vi "PXI-6229Loop.vi"(8 "Error In":errorcluster, 9 "ABLE Configuration":T1, 10 "PXI-6229 Data Notifier":refnum<notifier>, 11 "PXI-6229 Action Queue":refnum<queue>) -> (0 "Error Out":errorcluster)   [LabVIEW 2012]
uses:
  PXI6229ActionQueueElement.ctl
  PXI6229Action.ctl
  ABLEConfiguration.ctl
  DisplayConfiguration.ctl
  FolderConfiguration.ctl
  AlarmsConfiguration.ctl
  Keithley6485Configuration.ctl
  Keithley6482Configuration.ctl
  PXI6229Data.ctl
  <vilib>/Utility/error.llb/DialogType.ctl
  libs/LV-Utilities/LV-Utilities.lvlib
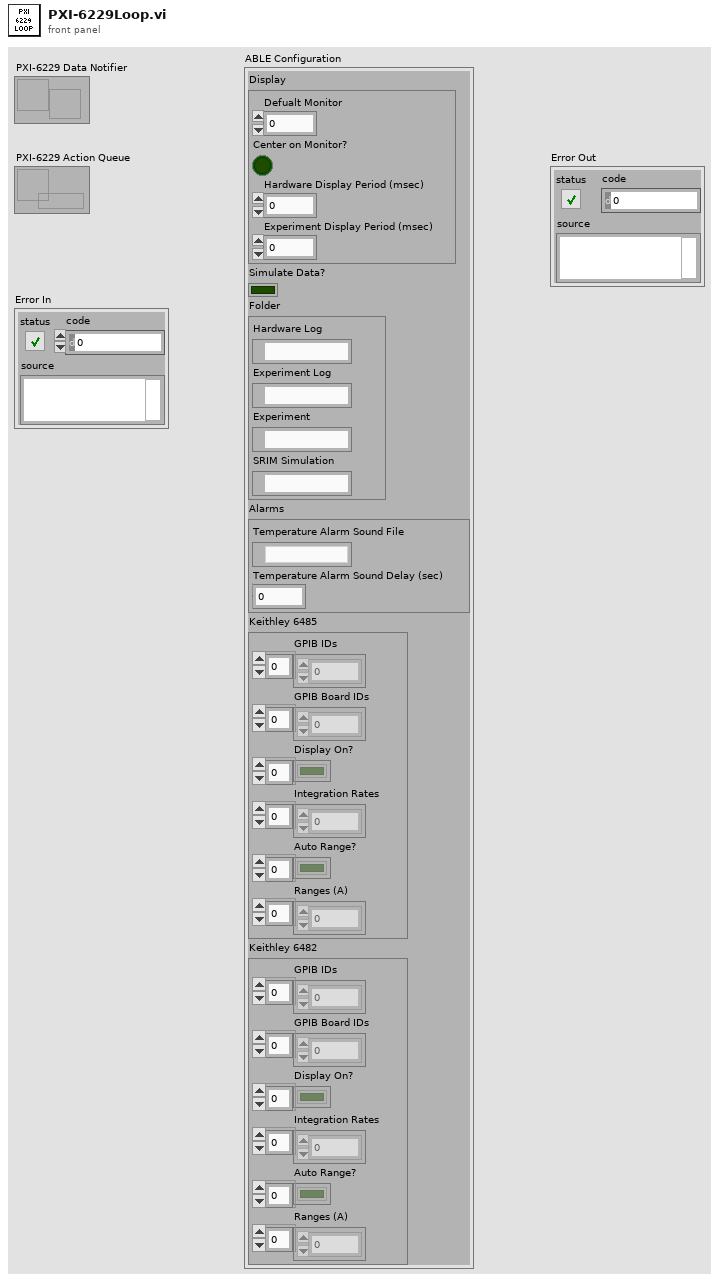
[diagram p1: front panel]
types:
  T1 = typedef "ABLEConfiguration.ctl" = cluster{"Display":T2, "Simulate Data?":bool, "Folder":T3, "Alarms":T4, "Keithley 6485":T5, "Keithley 6482":T6}
  T2 = typedef "DisplayConfiguration.ctl" = cluster{"Defualt Monitor":u16, "Center on Monitor?":bool, "Hardware Display Period (msec)":u32, "Experiment Display Period (msec)":u32}
  T3 = typedef "FolderConfiguration.ctl" = cluster{"Hardware Log":path, "Experiment Log":path, "Experiment":path, "SRIM Simulation":path}
  T4 = typedef "AlarmsConfiguration.ctl" = cluster{"Temperature Alarm Sound File":path, "Temperature Alarm Sound Delay (sec)":dbl}
  T5 = typedef "Keithley6485Configuration.ctl" = cluster{"GPIB IDs":u8[], "GPIB Board IDs":u8[], "Display On?":bool[], "Integration Rates":dbl[], "Auto Range?":bool[], "Ranges (A)":dbl[]}
  T6 = typedef "Keithley6482Configuration.ctl" = cluster{"GPIB IDs":u8[], "GPIB Board IDs":u8[], "Display On?":bool[], "Integration Rates":dbl[], "Auto Range?":bool[], "Ranges (A)":dbl[]}
  T7 = typedef "PXI6229Data.ctl" = cluster{"Temperatures":dbl[][], "Terminal Voltage":dbl[][], "BPM":dbl[][]}
  T8 = typedef "PXI6229ActionQueueElement.ctl" = cluster{"Action":T9, "Data":variant}
  T9 = typedef "PXI6229Action.ctl" = enum16{"Initialize", "Read", "Simulate", "Error", "Shutdown"}
  T10 = typedef "DialogType.ctl" = u16
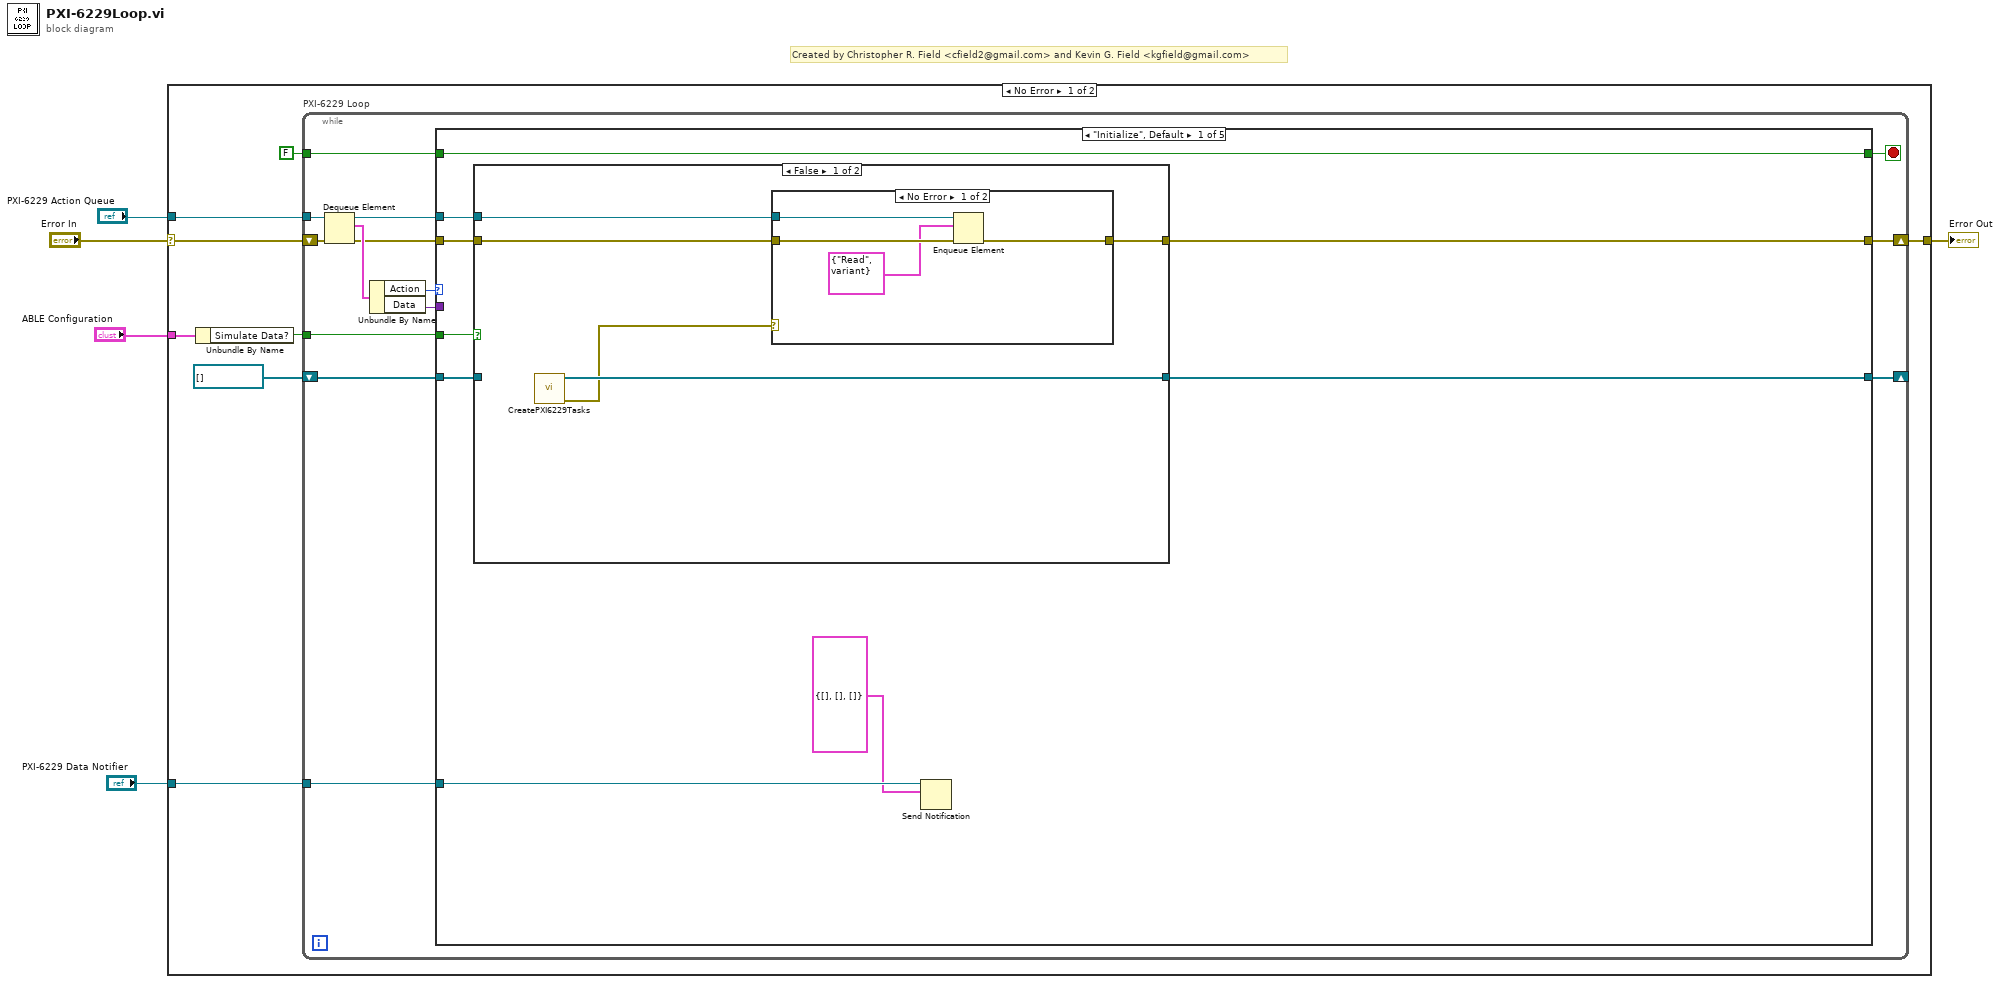
[diagram p0: block diagram]
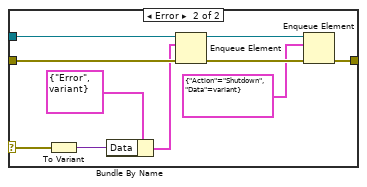
[diagram p2: hidden frame]
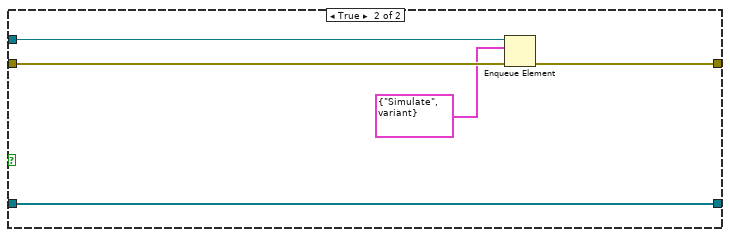
[diagram p3: hidden frame]
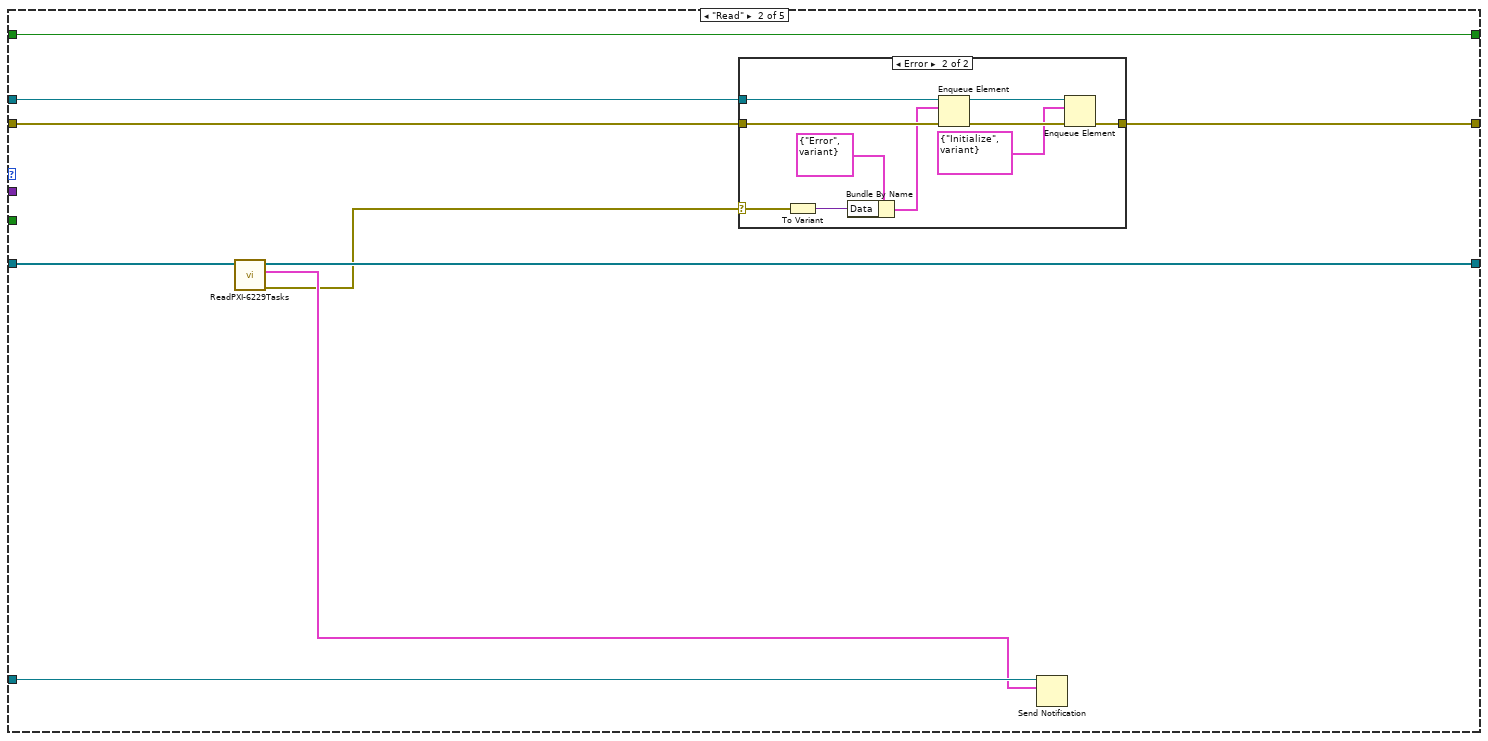
[diagram p4: hidden frame]
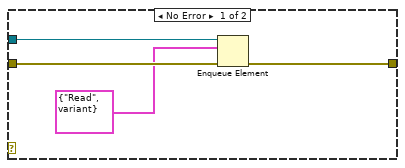
[diagram p5: hidden frame]
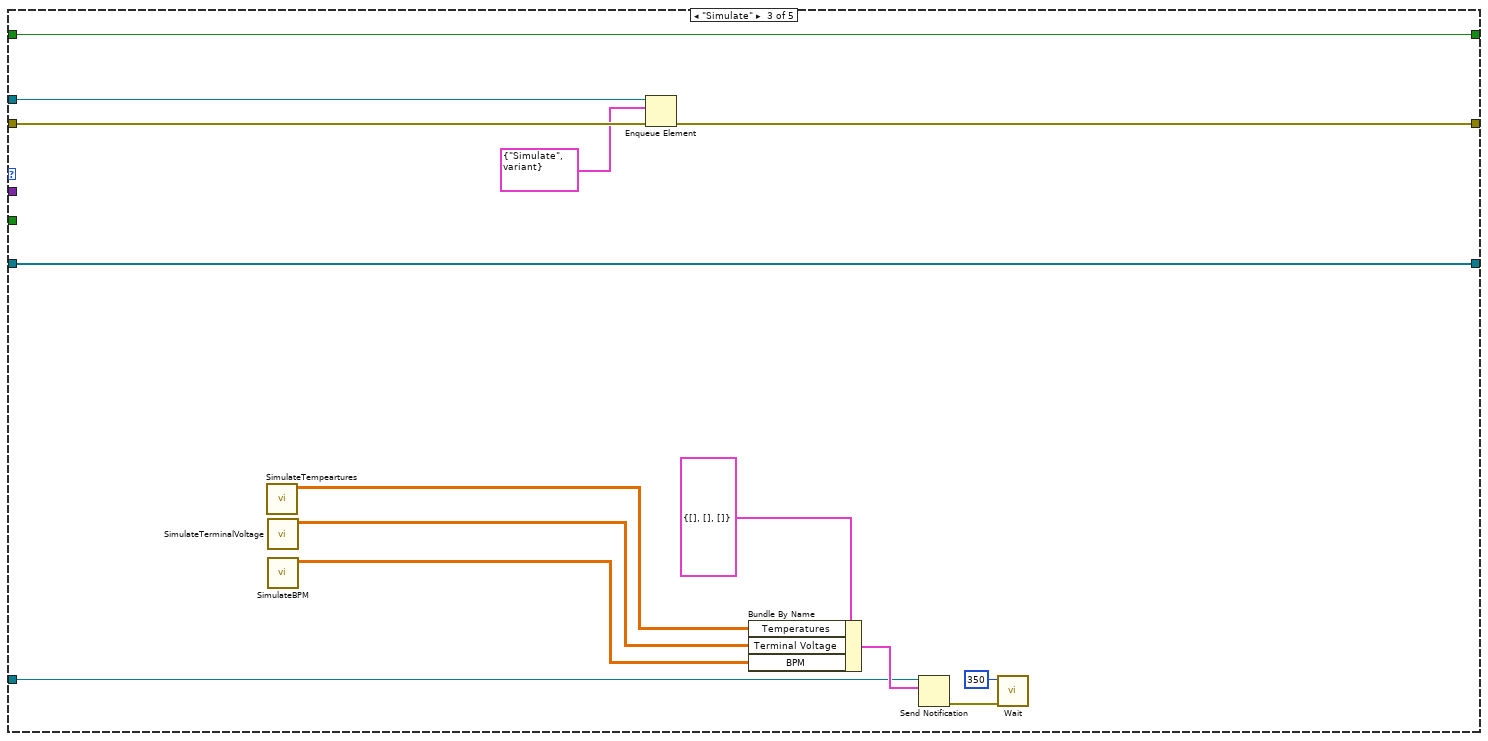
[diagram p6: hidden frame]
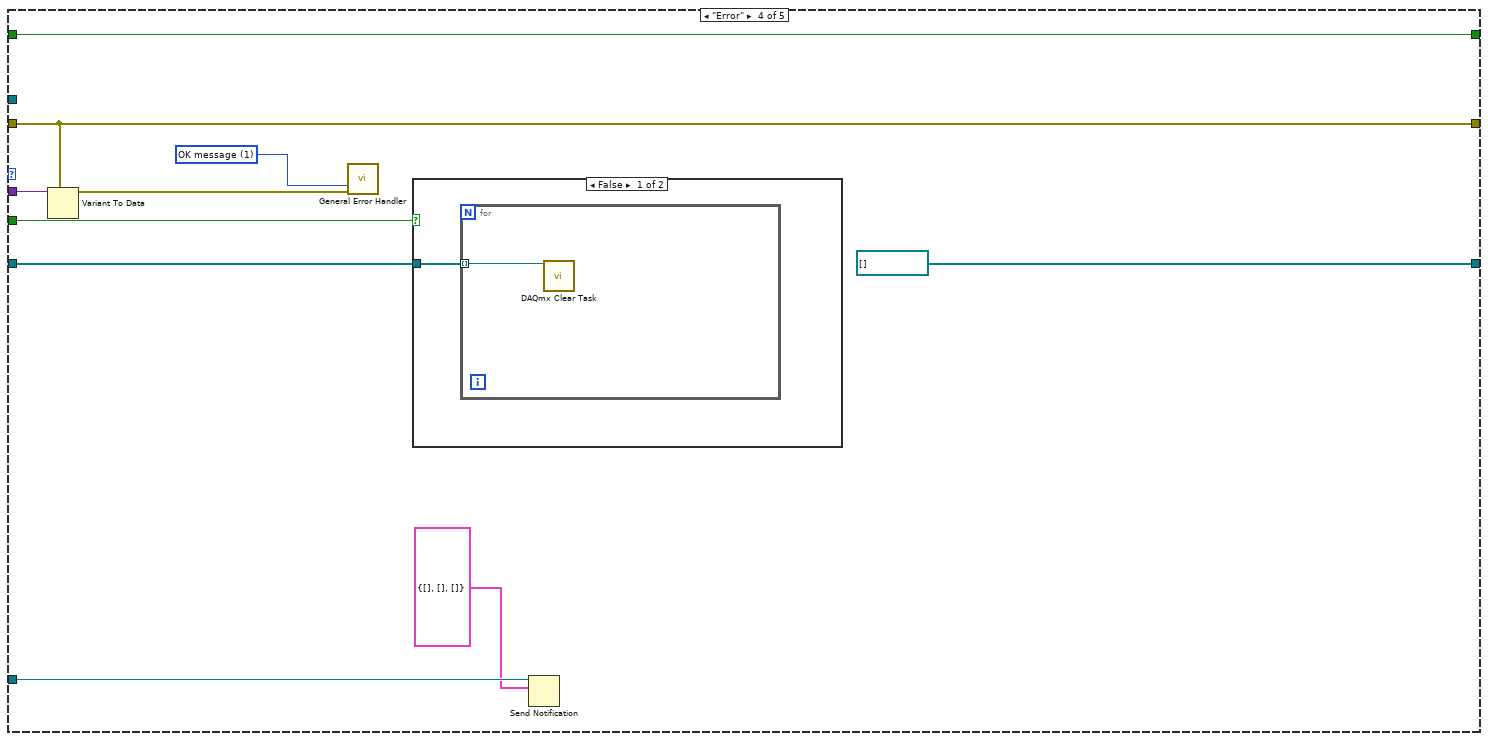
[diagram p7: hidden frame]
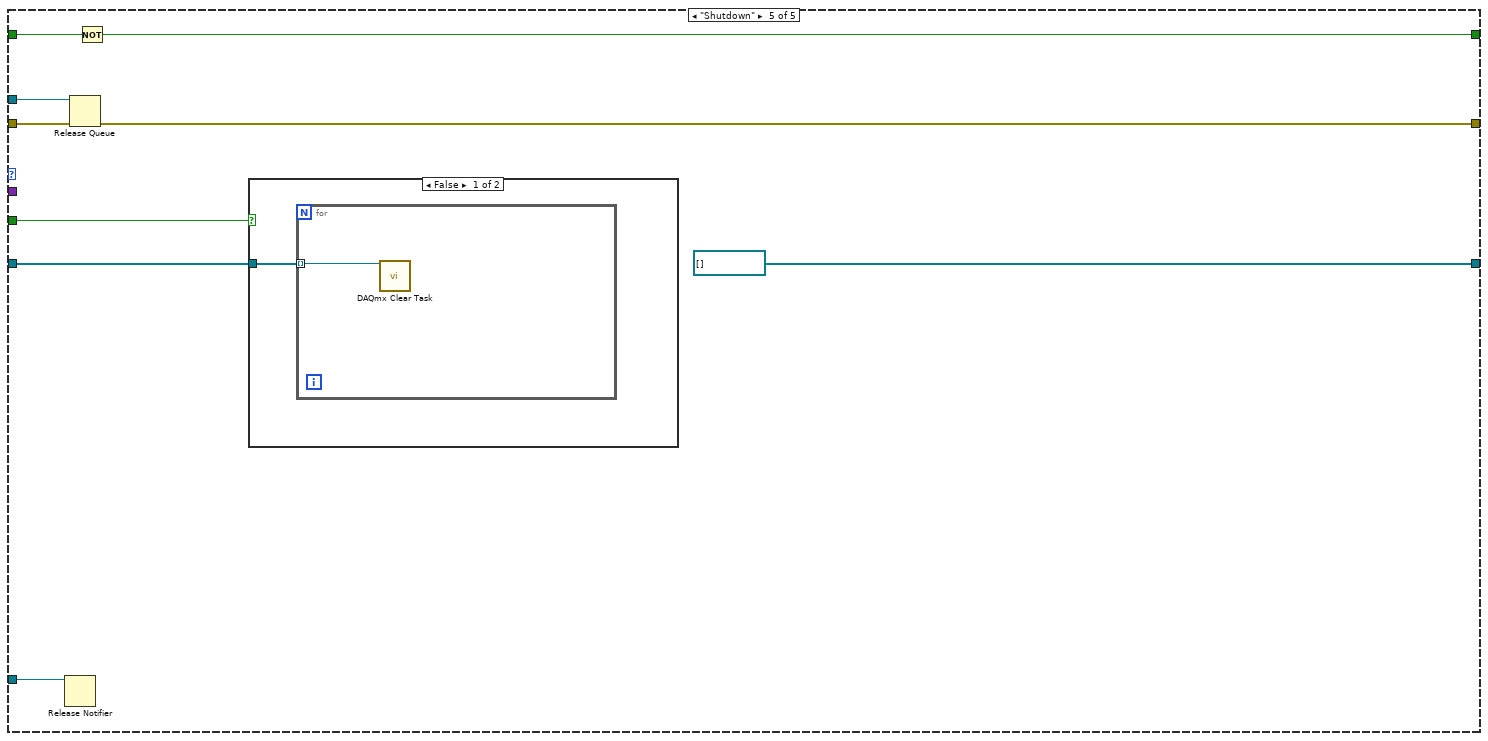
[diagram p9: hidden frame]
diagram:
  # "Created by Christopher R. Field <cfield2@gmail.com> and Kevin G. Field <kgfield@gmail.com>"
  n1 = case shown="No Error" "Error In" {
    selector: "Error In" -> [w10 w121]
    tunnel: "PXI-6229 Action Queue" -> [w13 _]
    tunnel: [w9 w121] -> w4
    tunnel: "PXI-6229 Data Notifier" -> [w11 _]
    tunnel: "ABLE Configuration" -> [w8 _]
    frame No Error {
      n2 = Unbundle By Name(w8) -> ("Simulate Data?"=w7:bool)
      n3 = while "PXI-6229 Loop" {
        tunnel: FALSE -> [w27]
        tunnel: w13 -> [w26]
        shift-right: [w18] -> w9
        shift-left: w10 -> [w25]
        tunnel: w11 -> [w17]
        shift-right: [w16] -> _
        shift-left: refnum<k21>[] [] -> [w15]
        tunnel: w7 -> [w14]
        stop <- w20 stop-if-true
        n4 = Dequeue Element(queue=w26, error in (no error)=w25) -> (queue out=w21:refnum<queue>, element=w24:T8, error out=w22:errorcluster)  [unwired: 1 in, 1 out]
        n5 = Unbundle By Name(w24) -> ("Action"=w23:T9, "Data"=w19:variant)
        n6 = case shown="\"Initialize\", Default" w23 {
          tunnel: w27 -> [w36 w69 w94 w107 w118]
          tunnel: w22 -> [w34 w66 w96 w103 w114]
          tunnel: w21 -> [w33 w68 w97 _ w116]
          tunnel: [w36 w69 w94 w107 w117] -> w20
          tunnel: w19 -> [_ _ _ w106 _]
          tunnel: [w32 w67 w95 w103 w115] -> w18
          tunnel: w17 -> [w29 w65 w89 w102 w111]
          tunnel: [w35 w63 w93 refnum<k21>[] [] ("PXI-6229 Tasks Out") refnum<k21>[] [] ("PXI-6229 Tasks Out")] -> w16
          tunnel: w15 -> [w30 w64 w93 w100 w113]
          tunnel: w14 -> [w31 _ _ w99 w112]
          frame "Initialize", Default {
            n7 = case shown="False" w31 {
              tunnel: [w38 w60] -> w35
              tunnel: w34 -> [w41 w58]
              tunnel: w33 -> [w40 w59]
              tunnel: [w39 w57] -> w32
              tunnel: w30 -> [_ w60]
              frame False {
                n8 = call "CreatePXI6229Tasks.vi"() -> ("Error Out"=w37:errorcluster, "PXI-6229 Tasks Out"=w38:refnum<k21>[])  [unwired: 10 in]
                n9 = case shown="No Error" w37 {
                  selector: w37 -> [_ w52]
                  tunnel: w41 -> [w44 w54]
                  tunnel: w40 -> [w45 w55]
                  tunnel: [w43 w47] -> w39
                  frame No Error {
                    n10 = Enqueue Element(queue=w45, element=T8 {"Action"=enum."Read", "Data"=variant}, error in (no error)=w44) -> (error out=w43:errorcluster)  [unwired: 1 in, 2 out]
                  }
                  frame Error {
                    n11 = To Variant(anything=w52) -> (Variant=w51:variant)
                    n12 = Bundle By Name(cluster=T8 {"Action"=enum."Error", "Data"=variant} ("element"), "Data"=w51) -> (w50:T8)
                    n13 = Enqueue Element(queue=w55, element=w50, error in (no error)=w54) -> (queue out=w49:refnum<queue>, error out=w48:errorcluster)  [unwired: 1 in, 1 out]
                    n14 = Enqueue Element(queue=w49, element=T8 {"Action"=enum."Shutdown", "Data"=variant}, error in (no error)=w48) -> (error out=w47:errorcluster)  [unwired: 1 in, 2 out]
                  }
                }
              }
              frame True {
                n15 = Enqueue Element(queue=w59, element=T8 {"Action"=enum."Simulate", "Data"=variant}, error in (no error)=w58) -> (error out=w57:errorcluster)  [unwired: 1 in, 2 out]
              }
            }
            n16 = Send Notification(notification=T7 {"Temperatures"=[], "Terminal Voltage"=[], "BPM"=[]}, notifier=w29) -> ()  [unwired: 1 in, 2 out]
          }
          frame "Read" {
            n17 = call "ReadPXI-6229Tasks.vi"("PXI-6229 Tasks In"=w64) -> ("Error Out"=w61:errorcluster, "PXI-6229 Data"=w62:T7, "PXI-6229 Tasks Out"=w63:refnum<k21>[])  [unwired: 8 in]
            n18 = case shown="Error" w61 {
              selector: w61 -> [_ w80]
              tunnel: w68 -> [w73 w83]
              tunnel: [w72 w75] -> w67
              tunnel: w66 -> [w71 w82]
              frame No Error {
                n19 = Enqueue Element(queue=w73, element=T8 {"Action"=enum."Read", "Data"=variant}, error in (no error)=w71) -> (error out=w72:errorcluster)  [unwired: 1 in, 2 out]
              }
              frame Error {
                n20 = To Variant(anything=w80) -> (Variant=w79:variant)
                n21 = Bundle By Name(cluster=T8 {"Action"=enum."Error", "Data"=variant} ("element"), "Data"=w79) -> (w78:T8)
                n22 = Enqueue Element(queue=w83, element=w78, error in (no error)=w82) -> (queue out=w77:refnum<queue>, error out=w76:errorcluster)  [unwired: 1 in, 1 out]
                n23 = Enqueue Element(queue=w77, element=T8 {"Action"=enum."Initialize", "Data"=variant}, error in (no error)=w76) -> (error out=w75:errorcluster)  [unwired: 1 in, 2 out]
              }
            }
            n24 = Send Notification(notification=w62, notifier=w65) -> ()  [unwired: 1 in, 2 out]
          }
          frame "Simulate" {
            n25 = call "SimulateTempeartures.vi"() -> ("Simulated Temperatures"=w84:dbl[][])  [unwired: 11 in]
            n26 = call "SimulateTerminalVoltage.vi"() -> ("Simulated Terminal Voltage"=w88:dbl[][])  [unwired: 11 in]
            n27 = call "SimulateBPM.vi"() -> ("Simulated BPM"=w87:dbl[][])  [unwired: 11 in]
            n28 = Enqueue Element(queue=w97, element=T8 {"Action"=enum."Simulate", "Data"=variant}, error in (no error)=w96) -> (error out=w95:errorcluster)  [unwired: 1 in, 2 out]
            n29 = Bundle By Name(cluster=T7 {"Temperatures"=[], "Terminal Voltage"=[], "BPM"=[]} ("DAQ Data Queue Element"), "Temperatures"=w84, "Terminal Voltage"=w88, "BPM"=w87) -> (w90:T7)
            n30 = Send Notification(notification=w90, notifier=w89) -> (error out=w85:errorcluster)  [unwired: 1 in, 1 out]
            n31 = call "Wait.vi"("Error In"=w85, "Wait Time (msec)"=u32 350) -> ()  [unwired: 9 in, 1 out]
          }
          frame "Error" {
            w104 = T10 1 items=["no dialog", "OK message", "continue or stop message", "OK message + warnings", "continue/stop + warnings"] ("type of dialog (OK msg:1)")
            n32 = Variant To Data(type=w103, Variant=w106) -> (data=w105:errorcluster)  [unwired: 1 in, 1 out]
            n33 = call <vilib>:"General Error Handler.vi"("type of dialog (OK msg:1)"=w104, "error in (no error)"=w105) -> ()  [unwired: 9 in, 5 out]
            n34 = case shown="False" w99 {
              tunnel: w100 -> [w108 _]
              frame False {
                n35 = for {
                  tunnel: w108 -> [w109] mode=indexing
                  n36 = call <vilib>:"DAQmx Clear Task.vi"("task in"=w109) -> ()  [unwired: 14 in, 1 out]
                }
              }
              frame True {
              }
            }
            n37 = Send Notification(notification=T7 {"Temperatures"=[], "Terminal Voltage"=[], "BPM"=[]}, notifier=w102) -> ()  [unwired: 1 in, 2 out]
          }
          frame "Shutdown" {
            n38 = Release Notifier(notifier=w111) -> ()  [unwired: 2 in, 3 out]
            n39 = Release Queue(queue=w116, error in (no error)=w114) -> (error out=w115:errorcluster)  [unwired: 1 in, 2 out]
            n40 = Not(x=w118) -> (.not. x?=w117:bool)
            n41 = case shown="False" w112 {
              tunnel: w113 -> [w119 _]
              frame False {
                n42 = for {
                  tunnel: w119 -> [w120] mode=indexing
                  n43 = call <vilib>:"DAQmx Clear Task.vi"("task in"=w120) -> ()  [unwired: 14 in, 1 out]
                }
              }
              frame True {
              }
            }
          }
        }
      }
    }
    frame Error {
    }
  }
  "Error Out" <- w4
